vi "example sending synchronous commands.vi"() -> ()   [LabVIEW 2016]
panel:
  in  "diff":i32
  in  "button 4":bool
  out "position":i32
  in  "button 3":bool
  out "known":T1(ring)
  in  "button 2":bool
  in  "button 1":bool
  in  "System Locator":string="usb:ix:0"
  out "Error":errorcluster
  in  "Steps":i32=1000 min=0 max=1000000 step=1
  in  "Amplitude":u32=4000 min=1 max=4000 step=1
  in  "Frequency":u32=8000 min=1 max=18500 step=1
  in  "stop":bool
  in  "Channel":u32
  out "System Index":u32
  in  "forward":bool
  in  "backward":bool
  in  "exit":bool
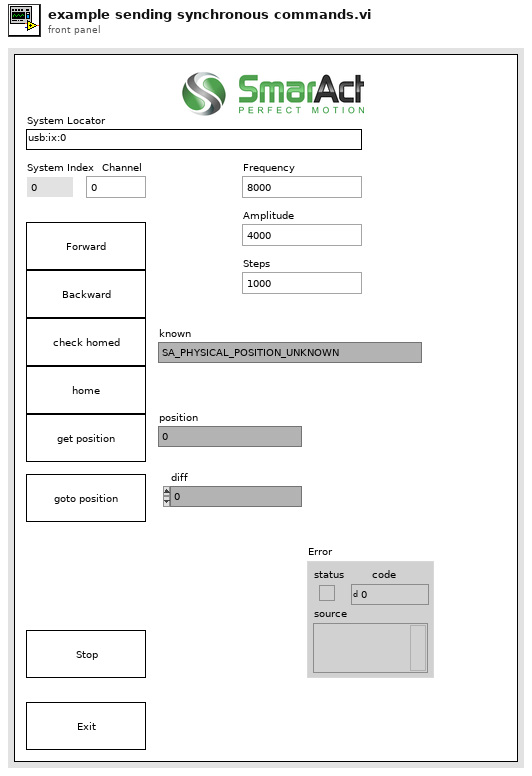
[diagram p1: front panel]
types:
  T1 = enum32{"SA_PHYSICAL_POSITION_UNKNOWN", "SA_PHYSICAL_POSITION_KNOWN"}
  T2 = enum32{"SA_FORWARD_DIRECTION", "SA_BACKWARD_DIRECTION", "SA_FORWARD_BACKWARD_DIRECTION", "SA_BACKWARD_FORWARD_DIRECTION"}
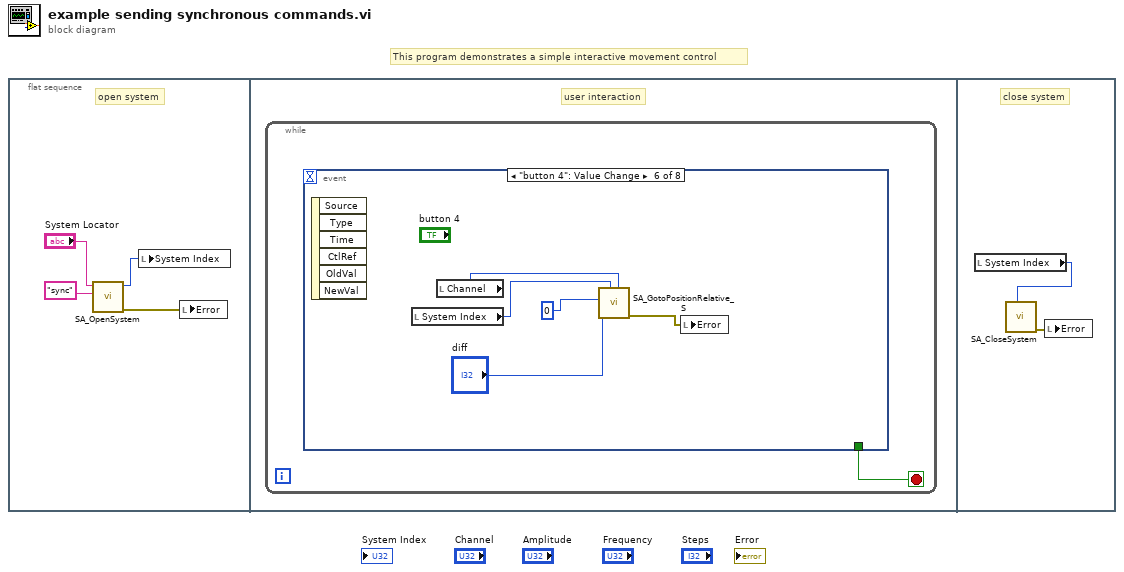
[diagram p0: block diagram]
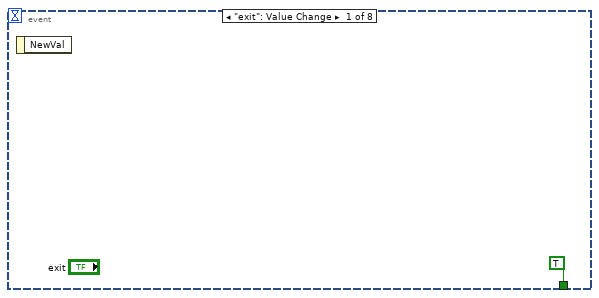
[diagram p2: hidden frame]
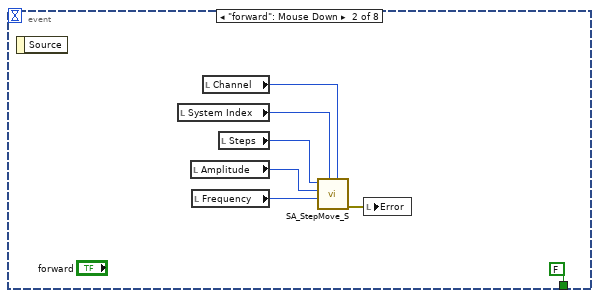
[diagram p3: hidden frame]
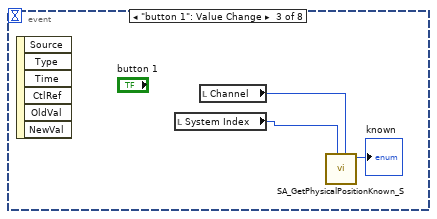
[diagram p4: hidden frame]
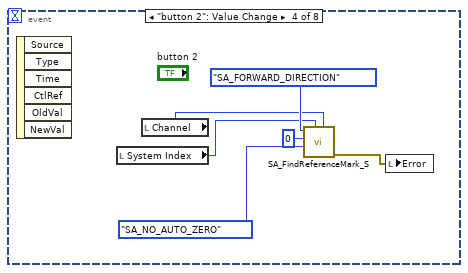
[diagram p5: hidden frame]
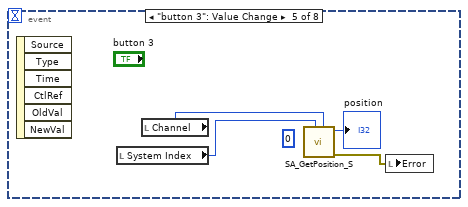
[diagram p6: hidden frame]
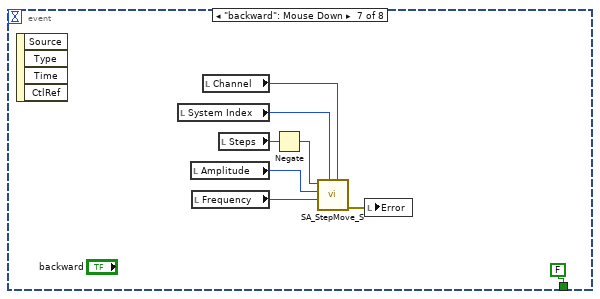
[diagram p7: hidden frame]
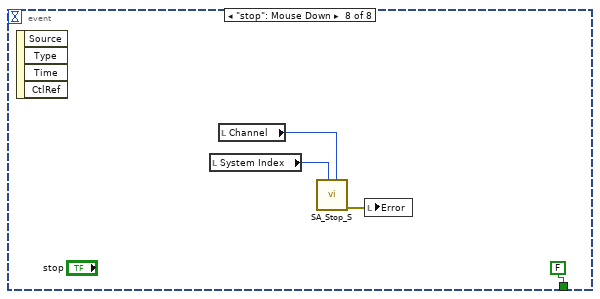
[diagram p8: hidden frame]
diagram:
  # "This program demonstrates a simple interactive movement control"
  n1 = flat-sequence {
    frame #0 {
      # "open system"
      n2 = call <vilib>:"SA_OpenSystem.vi"("options"="sync", "systemLocator"="System Locator") -> ("error out"=w4:errorcluster, "systemIndexOut"=w1:u32)  [unwired: 8 in]
      n3 = local write "System Index"(w1) -> ()
      n4 = local write "Error"(w4) -> ()
    }
    frame #1 {
      # "user interaction"
      n5 = while {
        stop <- w5 stop-if-true
        n6 = event shown="[5] \"button 4\": Value Change" {
          selector: _ -> [_ _ _ _ _ _ _ _]
          dyn-events: _ -> [_ _ _ _ _ _ _ _]
          timeout: _ -> [_ _ _ _ _ _ _ _]
          tunnel: [TRUE ("exit") FALSE ("exit") _ _ _ _ FALSE ("exit") FALSE ("exit")] -> w5
          event "exit": Value Change {
            n7 = event-data() -> ()  [unwired: 1 in, 1 out]
          }
          event "forward": Mouse Down {
            n8 = event-data() -> ()  [unwired: 1 in, 1 out]
            n9 = local read "System Index"() -> (w8:u32)
            n10 = local read "Amplitude"() -> (w9:u32)
            n11 = local read "Frequency"() -> (w10:u32)
            n12 = local read "Channel"() -> (w12:u32)
            n13 = local read "Steps"() -> (w11:i32)
            n14 = call <vilib>:"SA_StepMove_S.vi"("channelIndex"=w12, "systemIndex"=w8, "frequency"=w10, "amplitude"=w9, "steps"=w11) -> ("error out"=w7:errorcluster)  [unwired: 6 in]
            n15 = local write "Error"(w7) -> ()
          }
          event "button 1": Value Change {
            n16 = event-data() -> ()  [unwired: 1 in, 6 out]
            n17 = local read "System Index"() -> (w16:u32)
            n18 = local read "Channel"() -> (w15:u32)
            n19 = call <vilib>:"SA_GetPhysicalPositionKnown_S.vi"("channelIndex"=w15, "systemIndex"=w16) -> ("known"=→"known":T1)  [unwired: 8 in, 1 out]
          }
          event "button 2": Value Change {
            n20 = event-data() -> ()  [unwired: 1 in, 6 out]
            n21 = local read "System Index"() -> (w19:u32)
            n22 = local read "Channel"() -> (w18:u32)
            n23 = call <vilib>:"SA_FindReferenceMark_S.vi"("channelIndex"=w18, "systemIndex"=w19, "autoZero"=enum32{"SA_NO_AUTO_ZERO", "SA_AUTO_ZERO"}."SA_NO_AUTO_ZERO", "holdTime"=u32 0, "direction"=T2."SA_FORWARD_DIRECTION") -> ("error out"=w17:errorcluster)  [unwired: 6 in]
            n24 = local write "Error"(w17) -> ()
          }
          event "button 3": Value Change {
            (unwired) u32 0 ("holdTime")
            n25 = event-data() -> ()  [unwired: 1 in, 6 out]
            n26 = local read "System Index"() -> (w26:u32)
            n27 = local read "Channel"() -> (w25:u32)
            n28 = call <vilib>:"SA_GetPosition_S.vi"("channelIndex"=w25, "systemIndex"=w26) -> ("error out"=w24:errorcluster, "position"=→"position":i32)  [unwired: 8 in]
            n29 = local write "Error"(w24) -> ()
          }
          event "button 4": Value Change {
            n30 = event-data() -> ()  [unwired: 1 in, 6 out]
            n31 = local read "System Index"() -> (w31:u32)
            n32 = local read "Channel"() -> (w30:u32)
            n33 = call <vilib>:"SA_GotoPositionRelative_S.vi"("channelIndex"=w30, "systemIndex"=w31, "holdTime"=u32 0, "diff"="diff") -> ("error out"=w29:errorcluster)  [unwired: 7 in]
            n34 = local write "Error"(w29) -> ()
          }
          event "backward": Mouse Down {
            n35 = event-data() -> ()  [unwired: 1 in, 4 out]
            n36 = local read "System Index"() -> (w35:u32)
            n37 = local read "Amplitude"() -> (w36:u32)
            n38 = local read "Frequency"() -> (w37:u32)
            n39 = local read "Channel"() -> (w38:u32)
            n40 = local read "Steps"() -> (w33:i32)
            n41 = Negate(x=w33) -> (-x=w34:i32)
            n42 = call <vilib>:"SA_StepMove_S.vi"("channelIndex"=w38, "systemIndex"=w35, "frequency"=w37, "amplitude"=w36, "steps"=w34) -> ("error out"=w32:errorcluster)  [unwired: 6 in]
            n43 = local write "Error"(w32) -> ()
          }
          event "stop": Mouse Down {
            n44 = event-data() -> ()  [unwired: 1 in, 4 out]
            n45 = local read "System Index"() -> (w41:u32)
            n46 = local read "Channel"() -> (w42:u32)
            n47 = call <vilib>:"SA_Stop_S.vi"("channelIndex"=w42, "systemIndex"=w41) -> ("error out"=w40:errorcluster)  [unwired: 9 in]
            n48 = local write "Error"(w40) -> ()
          }
        }
      }
    }
    frame #2 {
      # "close system"
      n49 = local read "System Index"() -> (w44:u32)
      n50 = call <vilib>:"SA_CloseSystem.vi"("systemIndex"=w44) -> ("error out"=w45:errorcluster)  [unwired: 10 in]
      n51 = local write "Error"(w45) -> ()
    }
  }
